vi "Read write_.vi"(8 "error in (no error)":errorcluster, 11 "Set Write Ringdowns CMD in":refnum<class "Set Write Ringdowns CMD.lvclass">) -> (0 "error out":errorcluster, 2 "write?":bool, 3 "Set Write Ringdowns CMD out":refnum<class "Set Write Ringdowns CMD.lvclass">)   [LabVIEW 2014, in "eCRDS Library.lvlib" / "Set Write Ringdowns CMD.lvclass"]
uses:
  Set Write Ringdowns CMD.lvclass
  Set Write Ringdowns CMD.lvclass/Set Write Ringdowns CMD.ctl
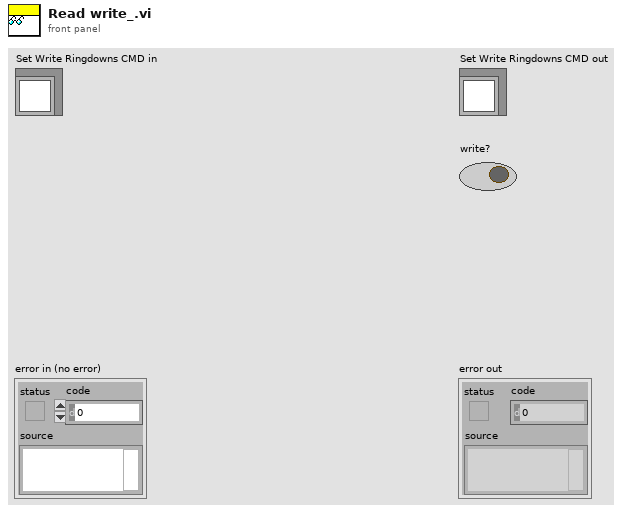
[diagram p1: front panel]
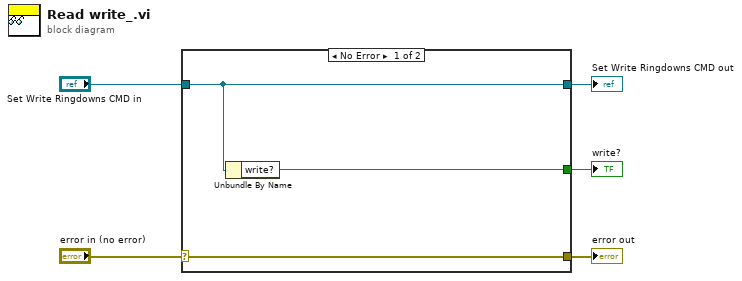
[diagram p0: block diagram]
diagram:
  n1 = case shown="No Error" "error in (no error)" {
    selector: "error in (no error)" -> [w8 w9]
    tunnel: [w8 w9] -> w4
    tunnel: [w7 w10] -> w2
    tunnel: "Set Write Ringdowns CMD in" -> [w7 w10]
    tunnel: [w6 _] -> w1
    frame No Error {
      n2 = Unbundle By Name(w7) -> ("write?"=w6:bool)
    }
    frame Error {
    }
  }
  "error out" <- w4
  "Set Write Ringdowns CMD out" <- w2
  "write?" <- w1
